vi "Status Updated.vi"(8 "error in (no error)":errorcluster, 10 "Status":string) -> (0 "error out":errorcluster)   [LabVIEW 2020, in "Settings Editor.lvlib"]
doc: "Send the Status Updated event to any VI registered to listen to events from the owning module.\n_____\nBased on Delacor QMH Project Template 4.0.0.47.\n_____\nBased on DQMH Project Template 6.0.0.91."
uses:
  Settings Editor.lvlib
  Status Updated Argument--cluster.ctl
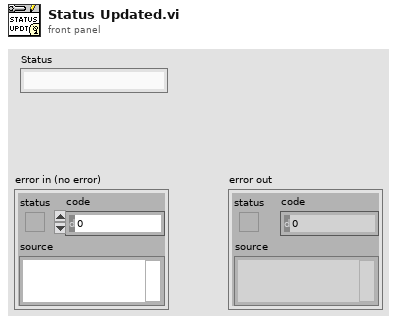
[diagram p1: front panel]
types:
  T1 = typedef "Settings Editor.lvlib/Status Updated Argument--cluster.ctl" = cluster{"Status":string}
  T2 = typedef "Settings Editor.lvlib/Broadcast Events--cluster.ctl" = cluster{"Module Did Init":refnum<user-event>, "Status Updated":refnum<user-event>, "Error Reported":refnum<user-event>, "Module Did Stop":refnum<user-event>, "Update Module Execution Status":refnum<user-event>, "Application Settings Updated":refnum<user-event>}
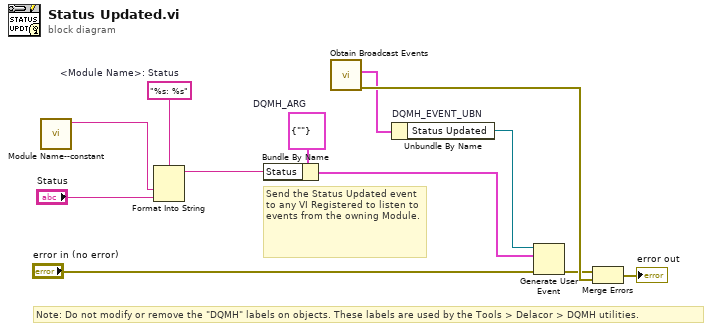
[diagram p0: block diagram]
diagram:
  w1 = "%s: %s"  # <Module Name>: Status
  w6 = T1 {"Status"=""}  # DQMH_ARG
  # "Note: Do not modify or remove the \"DQMH\" labels on objects. These labels are used by the Tools > Delacor > DQMH utilities."
  # "Send the Status Updated event to any VI Registered to listen to events from the owning Module."
  n1 = call "Module Name--constant.vi"() -> ("Module Name"=w2:string)  [unwired: 11 in]
  n2 = Format Into String(format string=w1, w2, "Status") -> (resulting string=w4:string)  [unwired: 2 in, 1 out]
  n3 = Bundle By Name(cluster=w6, "Status"=w4) -> (w5:T1)
  n4 = call "Obtain Broadcast Events.vi"() -> ("error out"=w10:errorcluster, "Settings Editor Broadcast Events"=w8:T2)  [unwired: 10 in]
  n5 = Unbundle By Name "DQMH_EVENT_UBN"(w8) -> ("Status Updated"=w7:refnum<user-event>)
  n6 = Generate User Event(user event=w7, event data cluster=w5, error in="error in (no error)") -> (error out=w9:errorcluster)  [unwired: 1 in, 1 out]
  n7 = Merge Errors(w9, w10) -> (→"error out":errorcluster)
